vi "ParseDescribeDetails.vi"(4 "DescribeDataIn":string[](array[string])) -> (1 "DescribeData":string[][](array[string]))   [LabVIEW 2023]
doc: "*-----------------------------------------------------\n* Author: SWatts\n*\n* VI Description: PARSE response from DESCRIBE request\n* \n*\n* Error handling: All errors passed out\n*\n* Pre-condition: \n*\n* Post-condition: None\n*\n* Revision History:\n*\n* Rev Date Author Description \n* 01 30/04/2014 SWatts First issue\n*\n*-----------------------------------------------------"
panel:
  # "Output"
  # "Input"
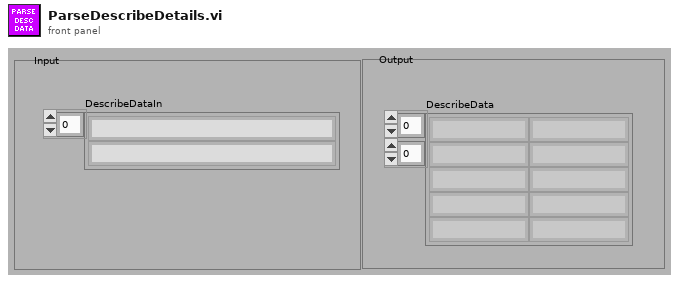
[diagram p1: front panel]
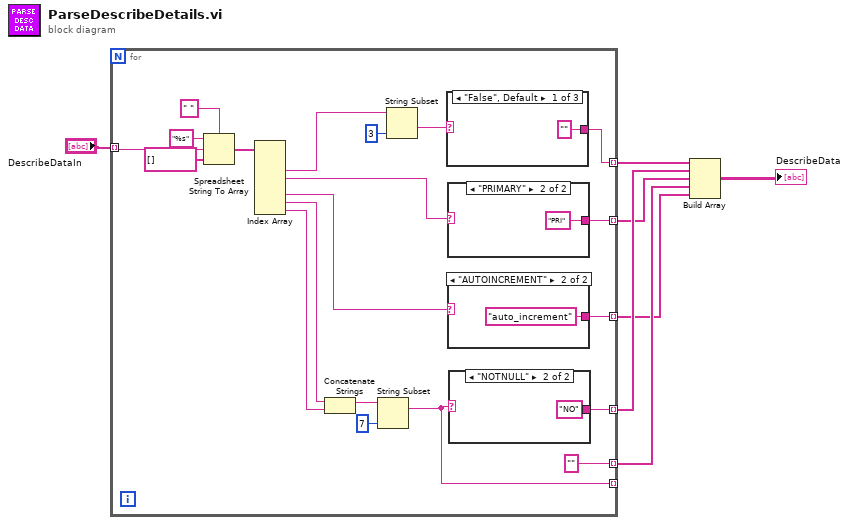
[diagram p0: block diagram]
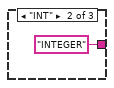
[diagram p2: hidden frame]
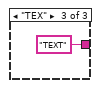
[diagram p3: hidden frame]
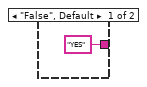
[diagram p4: hidden frame]
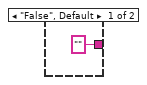
[diagram p5: hidden frame]
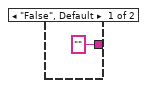
[diagram p6: hidden frame]
diagram:
  n1 = for {
    tunnel: "DescribeDataIn" -> [w27] mode=indexing
    tunnel: [w8] -> w6 mode=indexing
    tunnel: [w18] -> w5 mode=indexing
    tunnel: [w17] -> w4 mode=indexing
    tunnel: [w16] -> w2 mode=indexing
    tunnel: [""] -> w3 mode=indexing
    tunnel: [w12] -> _ mode=indexing
    n2 = Spreadsheet String To Array(delimiter (Tab)=" ", format string="%s", spreadsheet string=w27, array type (2D Dbl)=string[] []) -> (array=w23:string[])
    n3 = Index Array(array=w23) -> (element #2=w10:string, element #3=w22:string, element #5=w21:string, element #6=w20:string, element #7=w19:string)  [unwired: 7 in, 2 out]
    n4 = Concatenate Strings(w20, w19) -> (w14:string)
    n5 = String Subset(string=w14, length (rest)=7 ("length (rest)")) -> (substring=w12:string)  [unwired: 1 in]
    n6 = String Subset(string=w10, length (rest)=3 ("length (rest)")) -> (substring=w9:string)  [unwired: 1 in]
    n7 = case shown="\"False\", Default" w9 {
      tunnel: ["" "INTEGER" "TEXT"] -> w8
      frame "False", Default {
      }
      frame "INT" {
      }
      frame "TEX" {
      }
    }
    n8 = case shown="\"PRIMARY\"" w22 {
      tunnel: ["" "PRI"] -> w17
      frame "False", Default {
      }
      frame "PRIMARY" {
      }
    }
    n9 = case shown="\"AUTOINCREMENT\"" w21 {
      tunnel: ["" "auto_increment"] -> w16
      frame "False", Default {
      }
      frame "AUTOINCREMENT" {
      }
    }
    n10 = case shown="\"NOTNULL\"" w12 {
      tunnel: ["YES" "NO"] -> w18
      frame "False", Default {
      }
      frame "NOTNULL" {
      }
    }
  }
  n11 = Build Array(w6, w5, w4, w3, w2) -> (→"DescribeData":string[][])
